vi "FG_SignalStorage.vi"(7 "Command":T2=enum."Add_Signal", 8 "error in (no error)":errorcluster, 10 "SignalNumber":i32, 11 "DataIn":T1) -> (0 "error out":errorcluster, 3 "DataOut":T1, 4 "Signal_List":string[](array[string]))   [LabVIEW 2012]
uses:
  #TD_SignalStorageCommand.ctl
  #TD_SignalStorageData.ctl
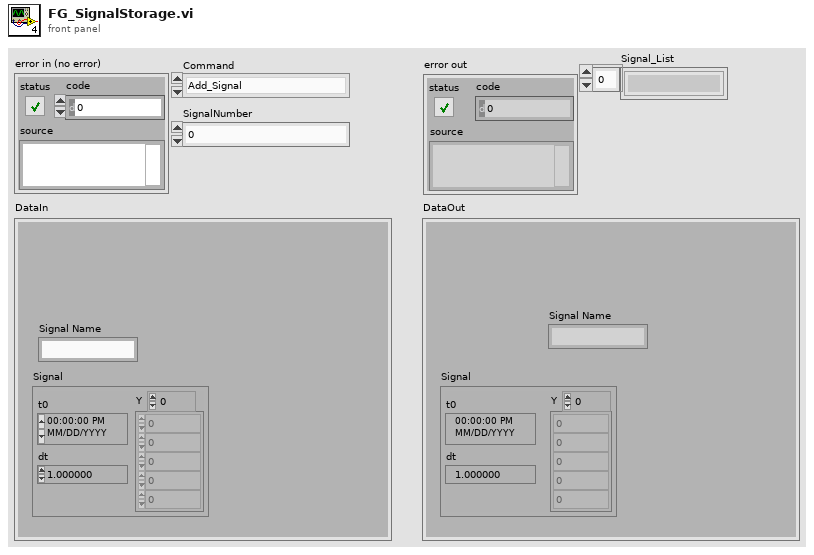
[diagram p1: front panel]
types:
  T1 = typedef "#TD_SignalStorageData.ctl" = cluster{"Signal":waveform(dbl), "Signal Name":string}
  T2 = typedef "#TD_SignalStorageCommand.ctl" = enum16{"Reset_Storage", "Add_Signal", "Insert_Signal", "Del_Signal", "Replace_Signal", "Get_Signal", "Get_Signal_List"}
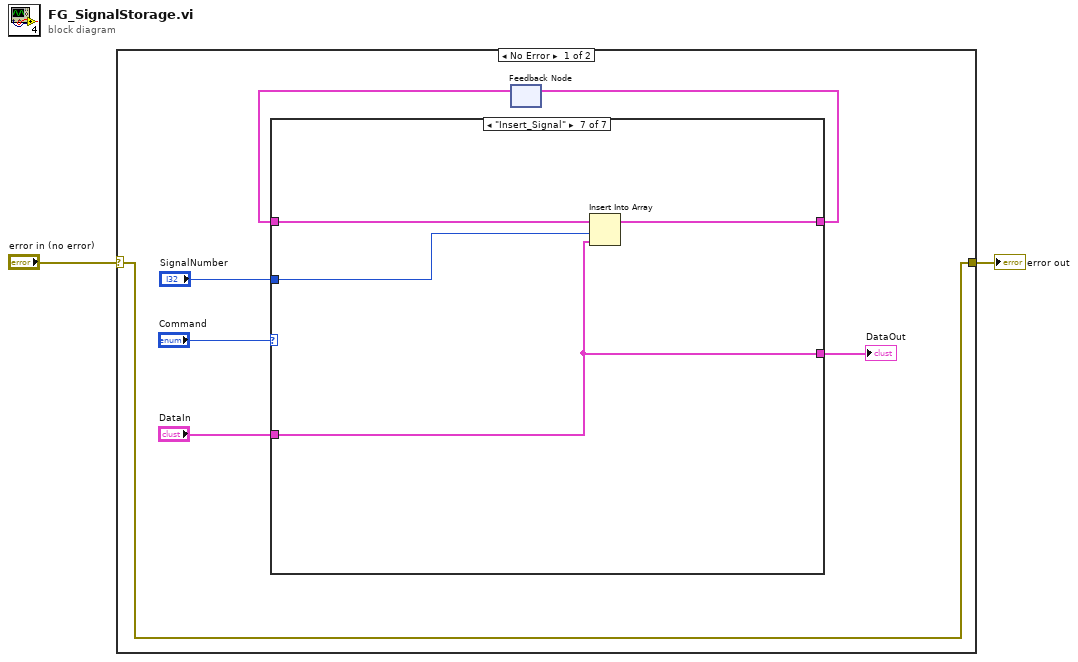
[diagram p0: block diagram]
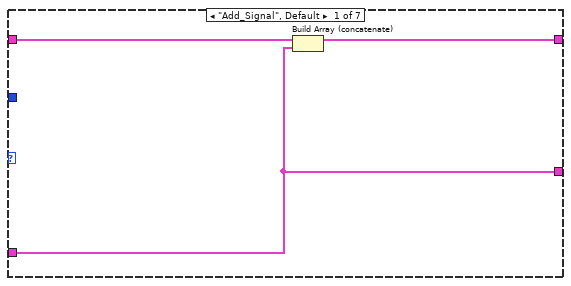
[diagram p2: hidden frame]
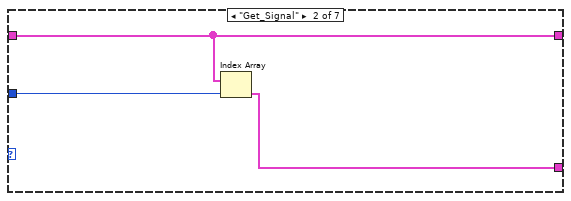
[diagram p3: hidden frame]
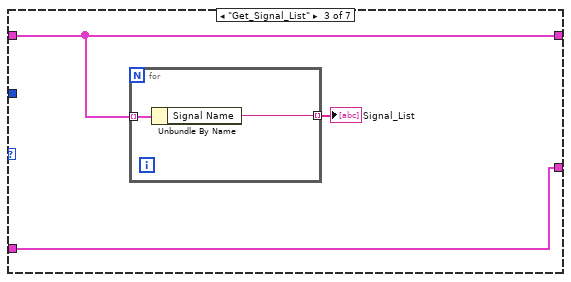
[diagram p4: hidden frame]
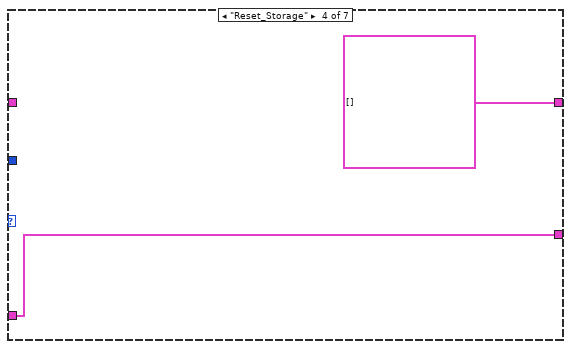
[diagram p5: hidden frame]
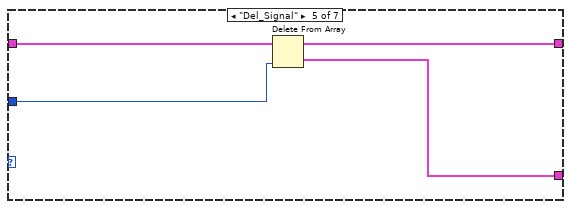
[diagram p6: hidden frame]
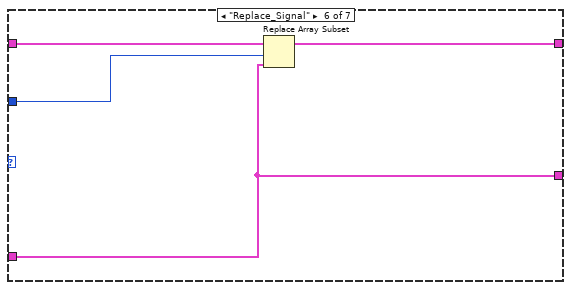
[diagram p7: hidden frame]
diagram:
  n1 = case shown="No Error" "error in (no error)" {
    selector: "error in (no error)" -> [w3 w35]
    tunnel: [w3 w35] -> w1
    frame No Error {
      n2 = feedback #1() -> (w6:T1[])  [unwired: 1 in]
      n3 = case shown="\"Insert_Signal\"" "Command" {
        tunnel: "DataIn" -> [w10 _ w16 w21 _ w27 w31]
        tunnel: [w12 w15 w18 T1[] [] ("appended array") w25 w29 w33] -> w7
        tunnel: w6 -> [w11 w15 w18 _ w26 w30 w34]
        tunnel: "SignalNumber" -> [_ w14 _ _ w24 w28 w32]
        tunnel: [w10 w13 w16 w21 w23 w27 w31] -> w4
        frame "Add_Signal", Default {
          n4 = Build Array (concatenate)(w11, w10) -> (w12:T1[])
        }
        frame "Get_Signal" {
          n5 = Index Array(array=w15, index=w14) -> (element=w13:T1)
        }
        frame "Get_Signal_List" {
          n6 = for {
            tunnel: w18 -> [w20] mode=indexing
            tunnel: [w19] -> w17 mode=indexing
            n7 = Unbundle By Name(w20) -> ("Signal Name"=w19:string)
          }
          "Signal_List" <- w17
        }
        frame "Reset_Storage" {
        }
        frame "Del_Signal" {
          n8 = Delete From Array(array=w26, index=w24) -> (deleted portion=w23:T1, array with subset deleted=w25:T1[])  [unwired: 1 in]
        }
        frame "Replace_Signal" {
          n9 = Replace Array Subset(array=w30, new element=w27, index=w28) -> (w29:T1[])
        }
        frame "Insert_Signal" {
          n10 = Insert Into Array(array=w34, index=w32, new element=w31) -> (w33:T1[])
        }
      }
      "DataOut" <- w4
      n11 = feedback-in #1(w7) -> ()
    }
    frame Error {
    }
  }
  "error out" <- w1
